vi "ExecutableInstance_core.vi"(11 "error in (no error)":errorcluster) -> (15 "error out":errorcluster)   [LabVIEW 2016, in "DronaTest.lvlib"]
uses:
  DronaTest.lvlib
  main/apis/Setup/GetVI/GetVIByName.vi
  <vilib>/addons/_JKI Toolkits/Caraya/classes/Assert/Assert Not Error.vi
  main/apis/Setup/GetVI/GetVI.lvlib
  <vilib>/addons/_JKI Toolkits/Caraya/classes/Assert/Assert.lvclass
  <vilib>/addons/_JKI Toolkits/Caraya/classes/Test/Test.lvclass
  main/Drona.lvlib
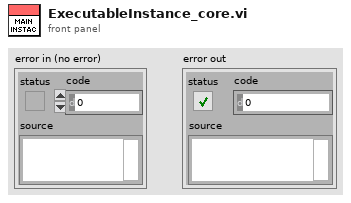
[diagram p1: front panel]
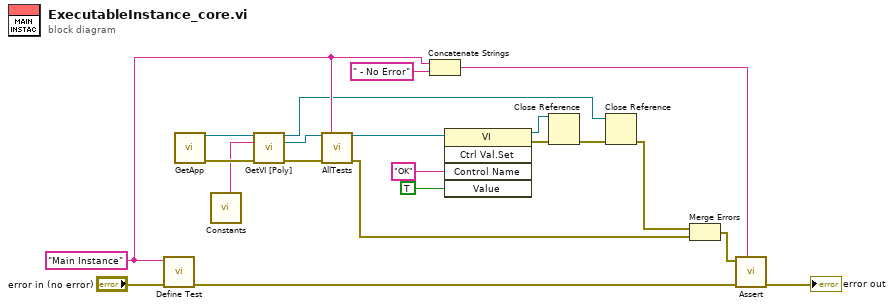
[diagram p0: block diagram]
diagram:
  w20 = "Main Instance" ("Label (VI Title)")
  n1 = call <vilib>:"Define Test.vi"("error in (no error)"="error in (no error)", "Label (VI Title)"=w20) -> ("error out"=w2:errorcluster)  [unwired: 9 in]
  n2 = call "GetApp.vi"() -> ("Application Ref"=w15:refnum<vi>, "error out"=w16:errorcluster)  [unwired: 14 in]
  n3 = call "Constants.vi"() -> ("HelperMain Name"=w14:string)  [unwired: 5 in, 6 out]
  n4 = call-poly "GetVI [Poly].vi"("Application Ref in"=w15, "VI Name"=w14, "error in (no error)"=w16) -> ("Application Ref out"=w4:refnum<vi>, "VI Reference"=w19:refnum<vi>, "error out"=w18:errorcluster)  [unwired: 10 in]
  n5 = call "AllTests.vi"("VI in"=w19, "Label"=w20, "error in (no error)"=w18) -> ("VI out"=w5:refnum<vi>, "error out"=w3:errorcluster)  [unwired: 11 in]
  n6 = Concatenate Strings(w20, " - No Error" ("Label (VI Title)")) -> (w6:string)
  n7 = invoke class="VI" method="Ctrl Val.Set"(reference=w5, "Control Name"="OK", "Value"=TRUE) -> (reference out=w12:refnum<vi>, error out=w13:errorcluster)  [unwired: 2 in, 3 out]
  n8 = Close Reference(reference=w12, error in (no error)=w13) -> (error out=w9:errorcluster)
  n9 = Close Reference(reference=w4, error in (no error)=w9) -> (error out=w7:errorcluster)
  n10 = Merge Errors(w7, w3) -> (w8:errorcluster)
  n11 = call-poly <vilib>:"Assert.vi"("Label"=w6, "error in (no error)"=w2, "Not Error?"=w8) -> ("error out"=→"error out":errorcluster)  [unwired: 8 in]
